vi "VINameUnescape.vi"(11 "escaped string":string) -> (3 "label":string)   [LabVIEW 2020]
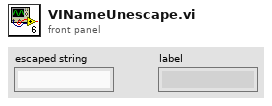
[diagram p1: front panel]
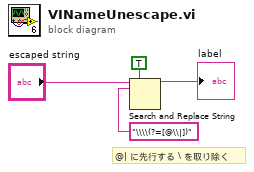
[diagram p0: block diagram]
diagram:
  # "@| に先行する \\ を取り除く"
  n1 = Search and Replace String(replace all?=TRUE ("replace all? (F)"), input string="escaped string", search string="\\\\(?=[@\\|])") -> (result string=→"label":string)  [unwired: 5 in, 3 out]
